vi "Test_NestedModelError_LogAndClearError_DoesNotStop.vi"(8 "error in (no error)":errorcluster, 11 "TestCase in":refnum<class "TestLaunchAndShutdown.lvclass">) -> (0 "error out":errorcluster, 3 "TestCase out":refnum<class "TestLaunchAndShutdown.lvclass">)   [LabVIEW 2020, in "TestLaunchAndShutdown.lvclass"]
uses:
  TestLaunchAndShutdown.lvclass
  TestLaunchAndShutdown.lvclass/TestLaunchAndShutdown.ctl
  24bf8875-c008-4f22-9bfa-88e42476d167.vi
  Source/IModel/IModel/IModel.lvclass
  <vilib>/ActorFramework/Actor/Actor.lvclass
  Source/Mediator/Mediator/Mediator.lvclass
  <vilib>/ActorFramework/Stop Msg/Stop Msg.lvclass
  modules/composed-event-logger/Source/String Control Sink/String Control Sink.lvclass
  modules/composed-event-logger/Source/Composed Log/Types/Log Level.ctl
  modules/composed-event-logger/Source/Composed Log/Composed Log.lvlib
  modules/composed-event-logger/Source/String Formats/String Expression Format/String Expression Format.lvclass
  Source/RootModel/RootModel/RootModel.lvclass
  Doubles/ModelLogsAndClearsErrors/ModelLogsAndClearsErrors.lvclass
  C:/Git/mva-core/Source/IModel/IModel/IModel.lvclass
  C:/Git/mva-core/Source/IObserver/IObserver/IObserver.lvclass
  C:/Program Files (x86)/National Instruments/LabVIEW 2020/vi.lib/ActorFramework/Actor/Actor.lvclass
  C:/Git/mva-core/Source/RootModel/RootModel/RootModel.lvclass
  0cab7304-49f4-4702-9b46-8e80122ef9d1.vi
  C:/Git/mva-core/modules/composed-event-logger/Source/IStringFormat/IStringFormat.lvclass
  C:/Git/mva-core/modules/composed-event-logger/Source/String Formats/String Expression Format/String Expression Format.lvclass
  C:/Git/mva-core/Test/Doubles/ModelGeneratesError/ModelGeneratesError.lvclass
  C:/Git/mva-core/Test/Doubles/ModelLogsAndClearsErrors/ModelLogsAndClearsErrors.lvclass
panel:
  in  "Full Log":string
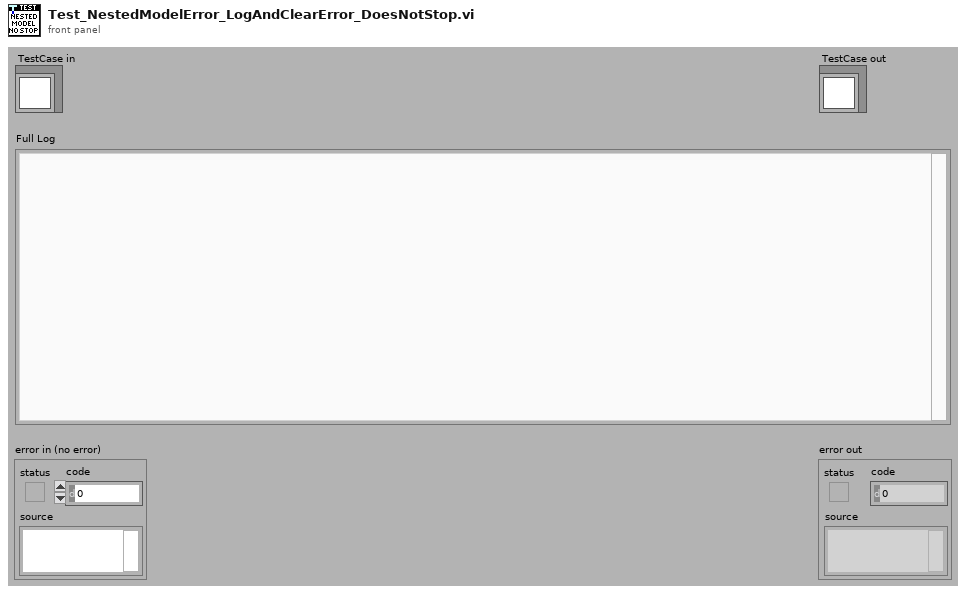
[diagram p1: front panel]
types:
  T1 = typedef "Composed Log.lvlib/Log Level.ctl" = enum16{"Debug", "Info", "Warning", "Error", "Critical"}
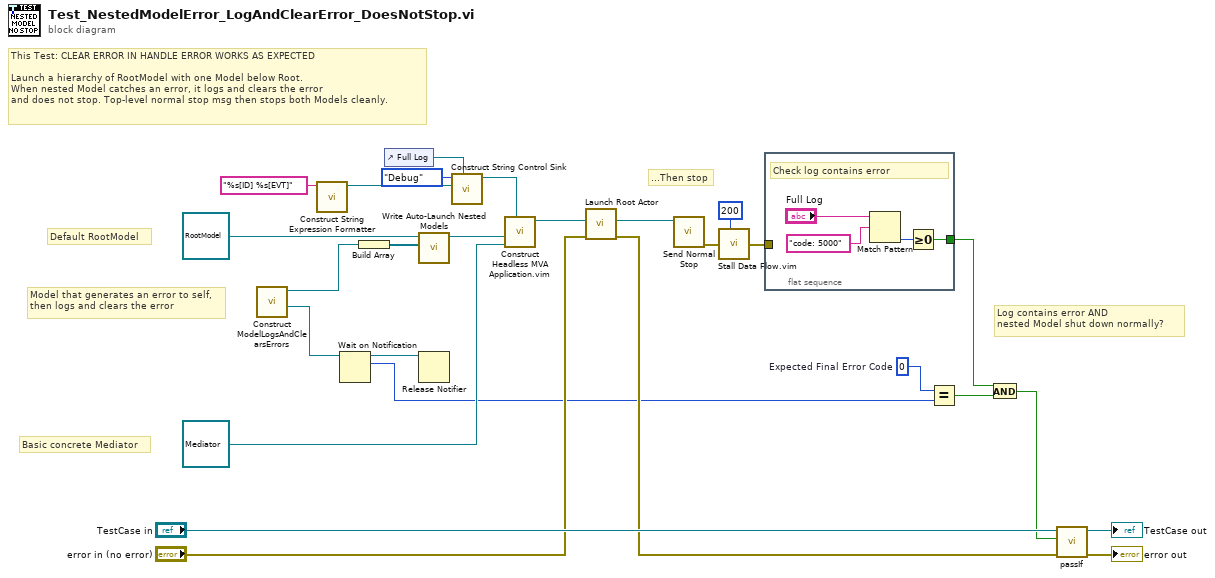
[diagram p0: block diagram]
diagram:
  w4 = 0  # Expected Final Error Code
  # "Log contains error AND\nnested Model shut down normally?"
  # "This Test: CLEAR ERROR IN HANDLE ERROR WORKS AS EXPECTED\n\nLaunch a hierarchy of RootModel with one Model below Root.\nWhen nested Model catches an error, it logs and clears the error\nand does not stop. Top-level normal stop msg then stops both Models cleanly."
  # "...Then stop"
  # "Model that generates an error to self,\nthen logs and clears the error"
  # "Default RootModel"
  # "Basic concrete Mediator"
  n1 = call "Construct ModelLogsAndClearsErrors.vi"() -> ("Final Error Notifier"=w11:refnum<notifier>, "ModelLogsAndClearsErrors out"=w12:refnum<class "ModelLogsAndClearsErrors.lvclass">)  [unwired: 10 in]
  n2 = call "Construct String Expression Formatter.vi"("Format Specifier"="%s[ID] %s[EVT]") -> ("String Expression Format out"=w16:refnum<class "String Expression Format.lvclass">)  [unwired: 9 in, 1 out]
  n3 = Wait on Notification(notifier=w11) -> (notifier out=w10:refnum<notifier>, notification=w5:i32)  [unwired: 3 in, 2 out]
  n4 = Build Array(w12) -> (w24:refnum<class "ModelLogsAndClearsErrors.lvclass">[])
  n5 = control-ref of="Full Log"() -> (w18:refnum<vi>)
  n6 = call "Write Auto-Launch Nested Models.vi"("Auto-Launch Nested Models"=w24, "IModel In"=refnum<class "RootModel.lvclass"> refnum ("RootModel.lvlib:RootModel.lvclass")) -> ("IModel Out"=w23:refnum<class "RootModel.lvclass">)  [unwired: 9 in]
  n7 = Release Notifier(notifier=w10) -> ()  [unwired: 2 in, 3 out]
  n8 = call "Construct String Control Sink.vi"("Str Refnum"=w18, "LogFormat"=w16, "LogLevel"=Log_Level."Debug") -> ("String Control Sink out"=w19:refnum<class "String Control Sink.lvclass">)  [unwired: 8 in]
  n9 = call "Construct Headless MVA Application.vim"("Event Log Sink(s)"=w19, "Mediator Type"=refnum<class "Mediator.lvclass"> refnum ("Mediator.lvlib:Mediator.lvclass"), "RootModel in"=w23) -> ("RootModel out"=w22:refnum<class "RootModel.lvclass">)  [unwired: 8 in]
  n10 = call <vilib>:"Launch Root Actor.vi"("error in (no error)"="error in (no error)", "Actor"=w22) -> ("error out"=w14:errorcluster, "Actor's Enqueuer"=w9:refnum<class "Message Enqueuer.lvclass">)  [unwired: 8 in]
  n11 = call <vilib>:"Send Normal Stop.vi"("Message Enqueuer"=w9) -> ("error out"=w8:errorcluster)  [unwired: 10 in]
  n12 = call "Stall Data Flow.vim"("value in"=w8, "milliseconds to wait"=u32 200) -> ("value out"=w7:errorcluster)  [unwired: 1 out]
  n13 = flat-sequence {
    tunnel: w7 -> [_]
    tunnel: [w28] -> w3
    frame #0 {
      # "Check log contains error"
      n14 = Match Pattern(string="Full Log", regular expression="code: 5000") -> (offset past match=w29:i32)  [unwired: 1 in, 3 out]
      n15 = Greater Or Equal To 0?(x=w29) -> (x >= 0?=w28:bool)
    }
  }
  n16 = Equal?(x=w4, y=w5) -> (x = y?=w2:bool)
  n17 = And(x=w3, y=w2) -> (x .and. y?=w1:bool)
  n18 = call-dynamic "passIf.vi"("error in (no error)"=w14, "pass"=w1, "TestCase in"="TestCase in") -> ("error out"=→"error out":errorcluster, "TestCase out"=→"TestCase out":refnum<class "TestLaunchAndShutdown.lvclass">)  [unwired: 7 in]
